vi "Main.vi"(11 "Module Admin":refnum<class "Delacor_lib_QMH_Module Admin.lvclass">) -> ()   [LabVIEW 2020, in "TCP_Server.lvlib"]
doc: "This template is based off of the Queued Message Handler design pattern and the Queued Message Handler project template that ships with LabVIEW.\n\nThe main difference is that the queue is private to this module and communication between modules is performed via Broadcast and Request events.\n\nRequest events are wrapped in public API methods and are handled in the Event Handling Loop (EHL) of this VI. Any module can register for Broadcast events sent by this module. The EHL generates messages based on user interface actions.\n\nThe Message Handling Loop (MHL) processes messages generated by the EHL, or by other messages. The messages are string values, so new messages can be added easily to the Message Cases case structure in the MHL. Each message cluster can also provide an optional value for Message Data, which is a variant that can be converted to whatever message-specific data is required.\n_____\nBased on DQMH Project Template 6.0.0.91."
uses:
  TCP_Server.lvlib
  <vilib>/Delacor/Delacor QMH/Libraries/Module Admin_class/Delacor_lib_QMH_Module Admin.lvclass
  Module Data--cluster.ctl
  <vilib>/Delacor/Delacor QMH/Libraries/Message Queue_class/Delacor_lib_QMH_Message Queue.lvclass/Delacor_lib_QMH_Message Queue.ctl
  Stop Argument--cluster.ctl
  <vilib>/Delacor/Delacor QMH/Libraries/Module Admin_class/Delacor_lib_QMH_Module Admin.lvclass/Delacor_lib_QMH_Module Admin.ctl
  <vilib>/Utility/miscctls.llb/LVPointTypeDef.ctl
  <vilib>/Delacor/Delacor QMH/Libraries/Message Queue_class/Delacor_lib_QMH_Enqueue Message (Single).vi
  <vilib>/Delacor/Delacor QMH/Libraries/Module Admin_class/Delacor_lib_QMH_Get External Launch.vi
  <vilib>/Utility/error.llb/Error Cluster From Error Code.vi
  <vilib>/ErrorRing/Error Ring.xnode
  <vilib>/Delacor/Delacor QMH/Libraries/Message Queue_class/Delacor_lib_QMH_Message Queue.lvclass
panel:
  out "concatenated string":string
  in  "Server":T1 {"Knob" scale=0.0..10.0; "Horizontal Fill Slide" scale=0.0..10.0}
  out "# of Connections":i32
  out "error out":errorcluster
  out "Status":string
  in  "Simulate MHL Error":bool
  in  "Simulate EHL Error":bool
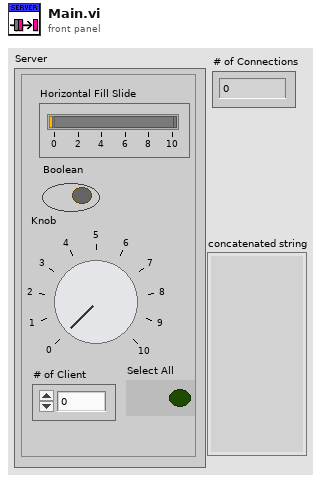
[diagram p1: front panel]
types:
  T1 = cluster{"Horizontal Fill Slide":dbl, "Knob":dbl, "Boolean":bool, "# of Client":i32, "Select All ":bool}
  T2 = typedef "TCP_Server.lvlib/Request Events--cluster.ctl" = cluster{"Stop Module":refnum<user-event>, "Show Panel":refnum<user-event>, "Hide Panel":refnum<user-event>, "Get Module Execution Status":refnum<user-event>, "Show Diagram":refnum<user-event>, "Wake Up HelperLoop":refnum<user-event>}
  T3 = typedef "TCP_Server.lvlib/Module Data--cluster.ctl" = cluster{"Status":string, "listener ID":refnum<k5>}
  T4 = enum32{"invalid lock state", "Not Locked", "Locked (No Password)", "Password-protected"}
  T5 = typedef "TCP_Server.lvlib/Stop Argument--cluster.ctl" = cluster{"Origin":string, "Exit via Stop Module Req?":bool, "Wait for Module to stop?":bool}
  T6 = typedef "LVPointTypeDef.ctl" = cluster{"Horizontal":i16, "Vertical":i16}
  T7 = enum32{"Invalid", "Standard", "Closed", "Hidden", "Minimized", "Maximized"}
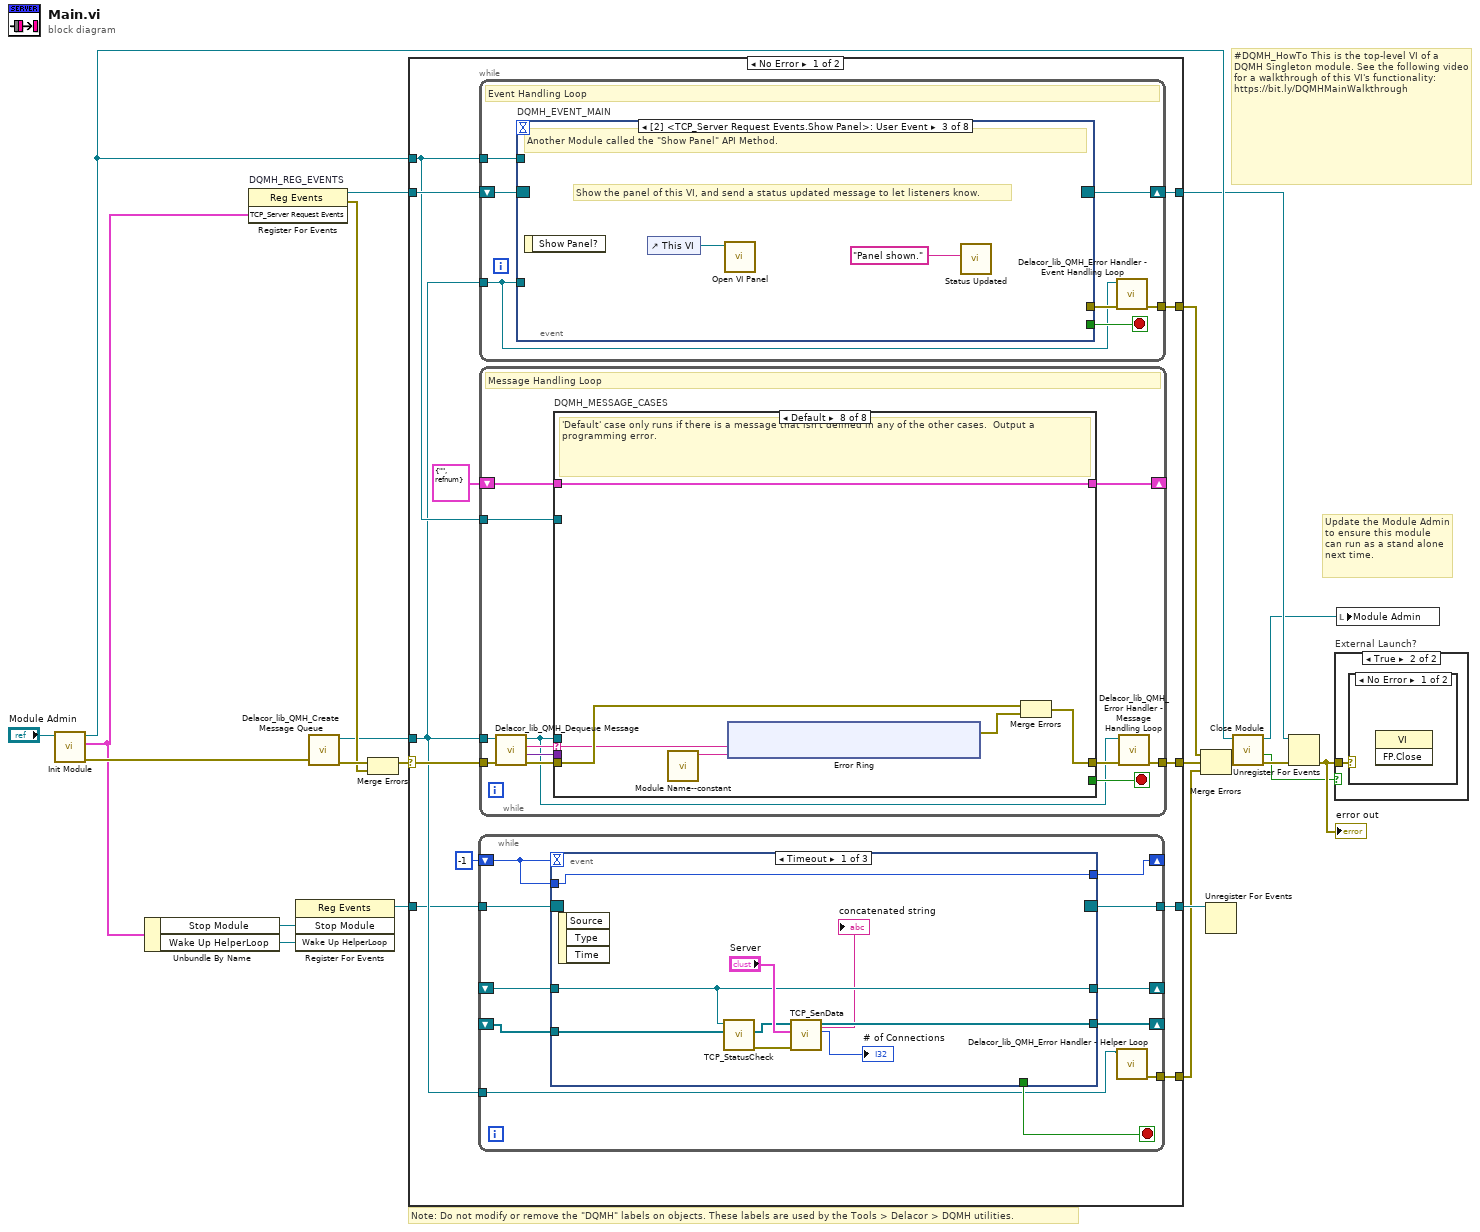
[diagram p0: block diagram]
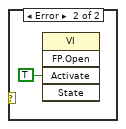
[diagram p3: hidden frame]
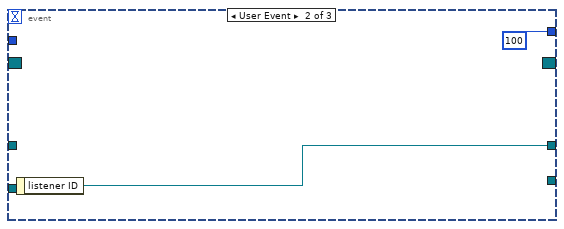
[diagram p4: hidden frame]
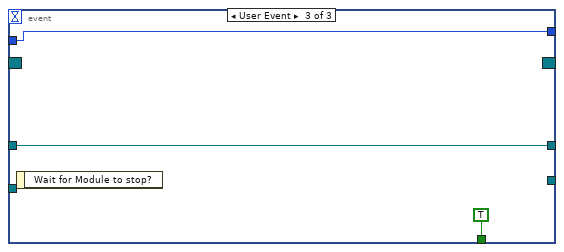
[diagram p5: hidden frame]
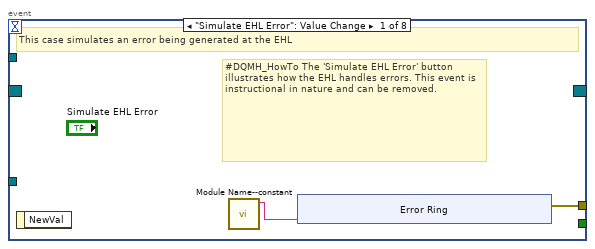
[diagram p6: hidden frame]
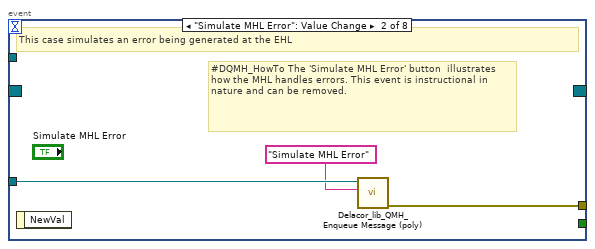
[diagram p7: hidden frame]
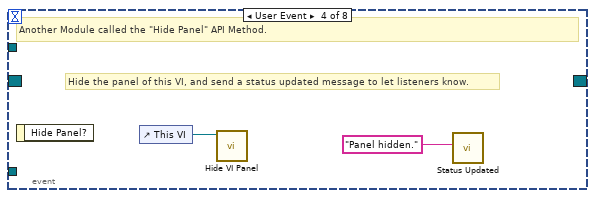
[diagram p8: hidden frame]
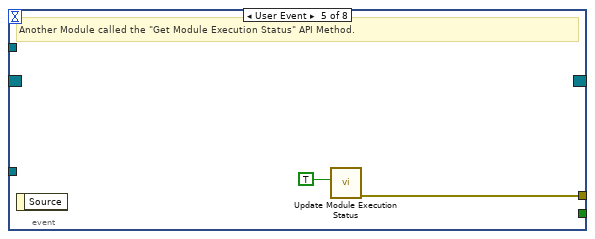
[diagram p9: hidden frame]
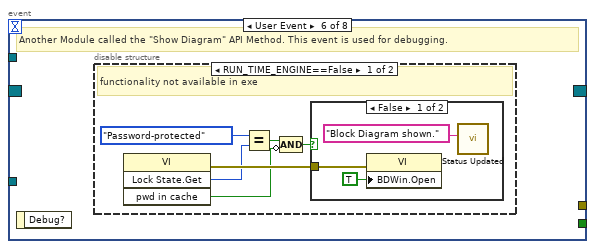
[diagram p10: hidden frame]
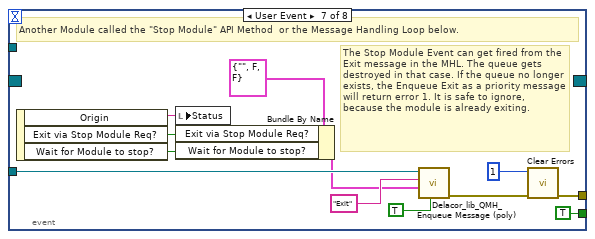
[diagram p13: hidden frame]
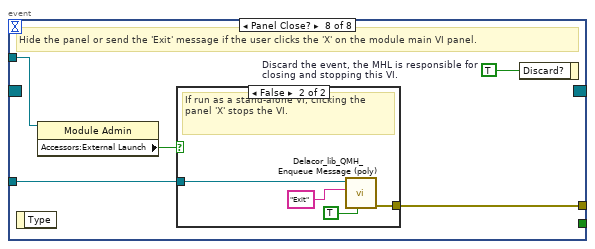
[diagram p14: hidden frame]
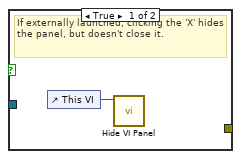
[diagram p15: hidden frame]
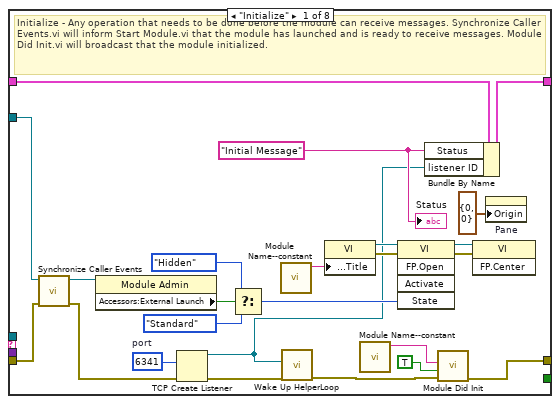
[diagram p16: hidden frame]
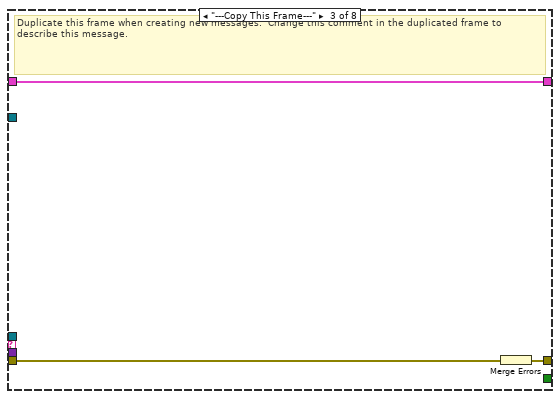
[diagram p18: hidden frame]
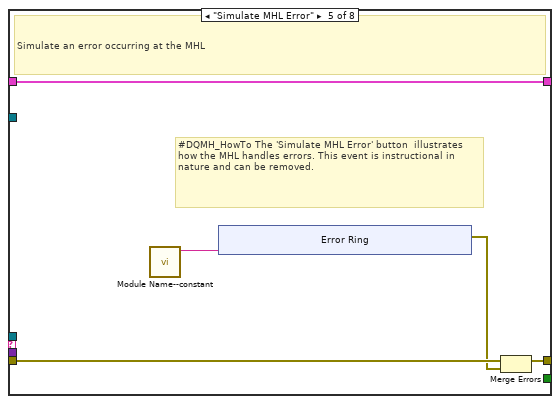
[diagram p20: hidden frame]
diagram:
  # "#DQMH_HowTo This is the top-level VI of a DQMH Singleton module. See the following video for a walkthrough of this VI's functionality: https://bit.ly/DQMHMainWalkthrough"
  # "Note: Do not modify or remove the \"DQMH\" labels on objects. These labels are used by the Tools > Delacor > DQMH utilities."
  # "Update the Module Admin to ensure this module can run as a stand alone next time."
  n1 = call "Init Module.vi"("Singleton Module Admin in"="Module Admin") -> ("error out"=w21:errorcluster, "TCP_Server Request Events"=w5:T2, "Singleton Module Admin out"=w13:refnum<class "Delacor_lib_QMH_Module Admin.lvclass">)  [unwired: 8 in]
  n2 = Unbundle By Name(w5) -> ("Stop Module"=w4:refnum<user-event>, "Wake Up HelperLoop"=w1:refnum<user-event>)
  n3 = register-events "DQMH_REG_EVENTS"(w5) -> (reference out=w11:refnum<event-registration>, error out=w14:errorcluster)  [unwired: 2 in]
  n4 = register-events(w4, w1) -> (reference out=w6:refnum<event-registration>)  [unwired: 2 in, 1 out]
  n5 = call <vilib>:"Delacor_lib_QMH_Create Message Queue.vi"("error in"=w21) -> ("error out"=w16:errorcluster, "Message Queue"=w10:refnum<class "Delacor_lib_QMH_Message Queue.lvclass">)  [unwired: 9 in]
  n6 = Merge Errors(w16, w14) -> (w15:errorcluster)
  n7 = case shown="No Error" w15 {
    selector: w15 -> [w32 w218]
    tunnel: [w34 w217] -> w22
    tunnel: [w31 w223] -> w12
    tunnel: w11 -> [w29 w223]
    tunnel: w10 -> [w27 w216]
    tunnel: [w33 _] -> w19
    tunnel: w13 -> [w28 w219]
    tunnel: w6 -> [w26 _]
    tunnel: [w24 _] -> w3
    tunnel: [w23 _] -> w2
    frame No Error {
      n8 = while {
        tunnel: w27 -> [w40]
        tunnel: w26 -> [w45]
        shift-right: [w43] -> _
        shift-left: -1 -> [w44]
        tunnel: [w42] -> w24
        tunnel: [w39] -> w23
        shift-right: [w38] -> _
        shift-left: _ -> [w37]
        shift-right: [w36] -> _
        shift-left: _ -> [w35]
        stop <- w41 stop-if-true
        n9 = event shown="[0] Timeout" {
          selector: w45 -> [_ _ _]
          dyn-events: [_ _ _] -> w42
          timeout: w44 -> [_ _ _]
          tunnel: w44 -> [w54 _ w57]
          tunnel: [w54 100 w57] -> w43
          tunnel: [_ _ TRUE] -> w41
          tunnel: [w47 w55 w58] -> w38
          tunnel: w37 -> [w47 _ w58]
          tunnel: [w52 _ _] -> w36
          tunnel: w35 -> [w48 _ _]
          event Timeout {
            n10 = event-data() -> ()  [unwired: 1 in, 3 out]
            n11 = call "TCP_StatusCheck.vi"("Clients"=w48, "listener ID in"=w47) -> ("no error"=w53:errorcluster, "Clients"=w49:refnum<k5>[])  [unwired: 7 in, 1 out]
            n12 = call "TCP_SenData.vi"("error in"=w53, "Server"="Server", "Clients"=w49) -> ("# of Connections"=→"# of Connections":i32, "Clients"=w52:refnum<k5>[], "concatenated string"=→"concatenated string":string)  [unwired: 4 in, 2 out]
          }
          event User Event {
            n13 = event-data() -> ("listener ID"=w55:refnum<k5>)  [unwired: 1 in]
          }
          event User Event {
            n14 = event-data() -> ()  [unwired: 1 in, 1 out]
          }
        }
        n15 = call-dynamic "Delacor_lib_QMH_Error Handler - Helper Loop.vi"("Message Queue in"=w40) -> ("dup error in"=w39:errorcluster)  [unwired: 9 in, 1 out]
      }
      n16 = while {
        tunnel: w27 -> [w60]
        shift-right: [w63] -> w31
        shift-left: w29 -> [w64]
        tunnel: [w65] -> w33
        tunnel: w28 -> [w61]
        stop <- w62 stop-if-true
        # "Event Handling Loop"
        n17 = event "DQMH_EVENT_MAIN" shown="[2] <TCP_Server Request Events.Show Panel>: User Event" {
          selector: w64 -> [_ _ _ _ _ _ _ _]
          dyn-events: [_ _ _ _ _ _ _ _] -> w63
          timeout: _ -> [_ _ _ _ _ _ _ _]
          tunnel: [_ _ _ _ _ _ TRUE ("Discard?") _] -> w62
          tunnel: w60 -> [_ w77 _ _ _ _ w101 w108]
          tunnel: [w68 w78 _ _ w84 _ w104 w110] -> w66
          tunnel: w61 -> [_ _ _ _ _ _ _ w107]
          event "Simulate EHL Error": Value Change {
            # "#DQMH_HowTo The 'Simulate EHL Error' button  illustrates how the EHL handles errors. This event is instructional in nature and can be removed."
            # "This case simulates an error being generated at the EHL"
            n18 = event-data() -> ()  [unwired: 1 in, 1 out]
            n19 = call "Module Name--constant.vi"() -> ("Module Name"=w67:string)  [unwired: 11 in]
            n20 = xnode "Error Ring"("parameter 0"=w67) -> ("error out"=w68:errorcluster)
          }
          event "Simulate MHL Error": Value Change {
            # "#DQMH_HowTo The 'Simulate MHL Error' button  illustrates how the MHL handles errors. This event is instructional in nature and can be removed."
            # "This case simulates an error being generated at the EHL"
            n21 = event-data() -> ()  [unwired: 1 in, 1 out]
            n22 = call-poly <vilib>:"Delacor_lib_QMH_Enqueue Message (poly).vi"("Message"="Simulate MHL Error", "Message Queue in"=w77) -> ("error out"=w78:errorcluster)  [unwired: 8 in, 1 out]
          }
          event User Event {
            # "Show the panel of this VI, and send a status updated message to let listeners know."
            # "Another Module called the \"Show Panel\" API Method."
            n23 = event-data() -> ()  [unwired: 1 in, 1 out]
            n24 = control-ref of="This VI"() -> (w80:refnum<vi>)
            n25 = call "Open VI Panel.vi"("VI"=w80) -> ()  [unwired: 10 in, 1 out]
            n26 = call "Status Updated.vi"("Status"="Panel shown." ("format string")) -> ()  [unwired: 10 in, 1 out]
          }
          event User Event {
            # "Hide the panel of this VI, and send a status updated message to let listeners know."
            # "Another Module called the \"Hide Panel\" API Method."
            n27 = event-data() -> ()  [unwired: 1 in, 1 out]
            n28 = control-ref of="This VI"() -> (w82:refnum<vi>)
            n29 = call "Hide VI Panel.vi"("VI"=w82) -> ()  [unwired: 10 in, 1 out]
            n30 = call "Status Updated.vi"("Status"="Panel hidden." ("format string")) -> ()  [unwired: 10 in, 1 out]
          }
          event User Event {
            # "Another Module called the \"Get Module Execution Status\" API Method."
            n31 = event-data() -> ()  [unwired: 1 in, 1 out]
            n32 = call "Update Module Execution Status.vi"("Running?"=TRUE) -> ("error out"=w84:errorcluster)  [unwired: 10 in]
          }
          event User Event {
            # "Another Module called the \"Show Diagram\" API Method. This event is used for debugging."
            n33 = event-data() -> ()  [unwired: 1 in, 1 out]
            n34 = disable-structure shown="RUN_TIME_ENGINE==False" {
              frame condition #0 (active) {
                # "functionality not available in exe"
                n35 = invoke class="VI" method="Lock State.Get"() -> (error out=w90:errorcluster, "Get Lock State"=w89:T4, "pwd in cache"=w86:bool)  [unwired: 4 in, 1 out]
                n36 = Equal?(x=T4."Password-protected", y=w89) -> (x = y?=w87:bool)
                n37 = Compound Arithmetic op=AND(w87, invert w86) -> (w85:bool)
                n38 = case shown="False" w85 {
                  tunnel: w90 -> [w93 _]
                  frame False {
                    n39 = property class="VI"(error in=w93, "BDWin.Open"=TRUE ("Block Diagram Window:Open")) -> ()  [unwired: 1 in, 2 out]
                    n40 = call "Status Updated.vi"("Status"="Block Diagram shown." ("format string")) -> ()  [unwired: 10 in, 1 out]
                  }
                  frame True {
                    # "Password-protected VI, and the password is not in the cache. Do not show the diagram."
                  }
                }
              }
              frame condition #1 {
              }
            }
          }
          event User Event {
            # "The Stop Module Event can get fired from the Exit message in the MHL. The queue gets destroyed in that case. If the queue no longer exists, the Enqueue Exit as a priority message will return error 1. It is safe to ignore, because the module is already exiting."
            # "Another Module called the \"Stop Module\" API Method  or the Message Handling Loop below."
            n41 = event-data() -> ("Origin"=w100:string, "Exit via Stop Module Req?"=w96:bool, "Wait for Module to stop?"=w95:bool)  [unwired: 1 in]
            n42 = local write "Status"(w100) -> ()
            n43 = Bundle By Name(cluster=T5 {"Origin"="", "Exit via Stop Module Req?"=FALSE, "Wait for Module to stop?"=FALSE} ("Stop Argument"), "Exit via Stop Module Req?"=w96, "Wait for Module to stop?"=w95) -> (w94:T5)
            n44 = call-poly <vilib>:"Delacor_lib_QMH_Enqueue Message (poly).vi"("Priority Message? (F)"=TRUE, "Message Data"=w94, "Message"="Exit", "Message Queue in"=w101) -> ("error out"=w105:errorcluster)  [unwired: 6 in, 1 out]
            n45 = call <vilib>:"Clear Errors.vi"("error in (no error)"=w105, "specific error code to clear (0: all)"=1) -> ("error out"=w104:errorcluster)  [unwired: 4 in, 1 out]
          }
          event Panel Close? {
            w109 = TRUE  # Discard the event, the MHL is responsible for closing and stopping this VI.
            # "Hide the panel or send the 'Exit' message if the user clicks the 'X' on the module main VI panel."
            n46 = event-data() -> ()  [unwired: 1 in, 1 out]
            n47 = property class="Module Admin"(reference=w107) -> ("Accessors:External Launch"=w106:bool)  [unwired: 1 in, 2 out]
            n48 = case shown="False" w106 {
              tunnel: w108 -> [_ w114]
              tunnel: [_ w115] -> w110
              frame True {
                # "If externally launched, clicking the 'X' hides the panel, but doesn't close it."
                n49 = control-ref of="This VI"() -> (w111:refnum<vi>)
                n50 = call "Hide VI Panel.vi"("VI"=w111) -> ()  [unwired: 10 in, 1 out]
              }
              frame False {
                # "If run as a stand-alone VI, clicking the panel 'X' stops the VI."
                n51 = call-poly <vilib>:"Delacor_lib_QMH_Enqueue Message (poly).vi"("Priority Message? (F)"=TRUE, "Message"="Exit", "Message Queue in"=w114) -> ("error out"=w115:errorcluster)  [unwired: 7 in, 1 out]
              }
            }
            n52 = event-data("Discard?"=w109) -> ()  [unwired: 1 in, 1 out]
          }
        }
        n53 = call-dynamic "Delacor_lib_QMH_Error Handler - Event Handling Loop.vi"("error in"=w66, "Message Queue in"=w60) -> ("dup error in"=w65:errorcluster)  [unwired: 8 in, 1 out]
      }
      n54 = while {
        tunnel: w27 -> [w118]
        shift-right: [w122] -> _
        shift-left: T3 {"Status"="", "listener ID"=refnum} ("Data Cluster") -> [w123]
        tunnel: w32 -> [w126]
        tunnel: [w124] -> w34
        tunnel: w28 -> [w116]
        stop <- w121 stop-if-true
        # "Message Handling Loop"
        n55 = call-dynamic "Delacor_lib_QMH_Dequeue Message.vi"("error in"=w126, "Message Queue in"=w118) -> ("error out"=w125:errorcluster, "Message Data"=w119:variant, "Message"=w120:string, "Message Queue out"=w117:refnum<class "Delacor_lib_QMH_Message Queue.lvclass">)  [unwired: 6 in]
        n56 = case "DQMH_MESSAGE_CASES" shown="Default" w120 {
          selector: w120 -> [_ _ _ _ _ _ _ w203]
          tunnel: w117 -> [_ _ _ _ _ w173 w195 _]
          tunnel: w125 -> [w149 w153 w156 w158 w163 w180 w201 w205]
          tunnel: [w148 w153 w155 w158 w162 w176 w198 w206] -> w127
          tunnel: w123 -> [w139 w152 w154 w157 w160 w175 w194 w204]
          tunnel: [w138 w152 w154 w157 w160 w175 w194 w204] -> w122
          tunnel: [_ _ _ _ _ _ w193 _] -> w121
          tunnel: w119 -> [_ _ _ _ _ w174 w192 _]
          tunnel: w116 -> [w140 _ _ _ _ w172 w187 _]
          frame "Initialize" {
            w131 = u16 6341  # port
            w134 = "Initial Message" ("Initial Message")
            # "Initialize - Any operation that needs to be done before the module can receive messages. Synchronize Caller Events.vi will inform Start Module.vi that the module has launched and is ready to receive messages. Module Did Init.vi will broadcast that the module initialized."
            n57 = call "Synchronize Caller Events.vi"("error in (no error)"=w149, "Singleton Module Admin in"=w140) -> ("error out"=w132:errorcluster, "Singleton Module Admin out"=w135:refnum<class "Delacor_lib_QMH_Module Admin.lvclass">)  [unwired: 8 in]
            n58 = property class="Module Admin"(reference=w135) -> ("Accessors:External Launch"=w144:bool)  [unwired: 1 in, 2 out]
            n59 = TCP Create Listener(8:w132, 10:w131) -> (0:w130:errorcluster, 3:w128:refnum<k5>)  [unwired: 1 in, 3 out]
            n60 = Select(t=T7."Hidden" ("State"), s=w144, f=T7."Standard" ("State")) -> (s? t:f=w141:T7)
            n61 = call "Module Name--constant.vi"() -> ("Module Name"=w147:string)  [unwired: 11 in]
            n62 = call "Wake Up HelperLoop.vi"("error in"=w130, "listener ID"=w128) -> ("error out"=w129:errorcluster)  [unwired: 9 in]
            n63 = property class="VI"("Front Panel.Title"=w147) -> (reference out=w146:refnum<vi>, error out=w151:errorcluster)  [unwired: 2 in]
            n64 = call "Module Name--constant.vi"() -> ("Module Name"=w136:string)  [unwired: 11 in]
            n65 = invoke class="VI" method="FP.Open"(reference=w146, error in=w151, "State"=w141) -> (reference out=w145:refnum<vi>, error out=w150:errorcluster)  [unwired: 2 in, 3 out]
            n66 = Bundle By Name(cluster=w139, "Status"=w134, "listener ID"=w128) -> (w138:T3)
            n67 = call "Module Did Init.vi"("error in (no error)"=w129, "Initialized?"=TRUE, "Origin"=w136) -> ("error out"=w148:errorcluster)  [unwired: 8 in]
            n68 = invoke class="VI" method="FP.Center"(reference=w145, error in=w150) -> ()  [unwired: 1 in, 3 out]
            n69 = property on="Pane" class="Pane"("Origin"=T6 {"Horizontal"=0, "Vertical"=0}) -> ()  [unwired: 2 in, 2 out]
            "Status" <- w134
          }
          frame "---Module Specific---" {
            # "Separator -- The following cases handle messages specific to this Module."
          }
          frame "---Copy This Frame---" {
            # "Duplicate this frame when creating new messages.  Change this comment in the duplicated frame to describe this message."
            n70 = Merge Errors(w156) -> (w155:errorcluster)
          }
          frame "---Exit and Error Handling---" {
            # "Separator - The following cases handle errors and exit messages."
          }
          frame "Simulate MHL Error" {
            # "#DQMH_HowTo The 'Simulate MHL Error' button  illustrates how the MHL handles errors. This event is instructional in nature and can be removed."
            # "Simulate an error occurring at the MHL"
            n71 = call "Module Name--constant.vi"() -> ("Module Name"=w159:string)  [unwired: 11 in]
            n72 = xnode "Error Ring"("parameter 0"=w159) -> ("error out"=w161:errorcluster)
            n73 = Merge Errors(w163, w161) -> (w162:errorcluster)
          }
          frame "Error" {
            # "#CodeRecommended - If you ever change the name of this \"Error\" message, you'll need to update the name in the Check Loop Error.vi as well."
            # "#CodeRecommended - If the module is running in standalone mode (External Launch = FALSE), this code will pop up an error dialog and call the 'Exit' message if an error occurs. Add more fine-grained error handling here."
            # "Error - Check the error message data and respond accordingly. This message is sent by the \"Error Handler\" VIs at the end of each loop in this application."
            n74 = property class="Module Admin"(reference=w172) -> ("Accessors:External Launch"=w171:bool)  [unwired: 1 in, 2 out]
            n75 = Variant To Data(error in=w180, type=errorcluster {"status"=FALSE, "code"=0, "source"=""} ("error constant"), Variant=w174) -> (data=w181:errorcluster, error out=w178:errorcluster)
            n76 = call "Error Reported.vi"("Error"=w181) -> ()  [unwired: 10 in, 1 out]
            n77 = case shown="False" w171 {
              tunnel: [w186 _] -> w177
              tunnel: w173 -> [w184 _]
              tunnel: w181 -> [w185 _]
              frame False {
                # "If the module is running standalone, then pop up an error dialog and call the \"Exit\" message."
                n78 = call <vilib>:"Simple Error Handler.vi"("error in (no error)"=w185) -> ()  [unwired: 4 in, 5 out]
                n79 = call-poly <vilib>:"Delacor_lib_QMH_Enqueue Message (poly).vi"("Priority Message? (F)"=TRUE, "Message"="Exit", "Message Queue in"=w184) -> ("error out"=w186:errorcluster)  [unwired: 7 in, 1 out]
              }
              frame True {
                # "If the module was launched externally, calling the Error Reported broadcast VI is the only action performed by the \"Error\" message. The module's caller can then process the error appropriately."
              }
            }
            n80 = Merge Errors(w178, w177) -> (w176:errorcluster)
            n81 = local write "error out"(w176) -> ()
          }
          frame "Exit" {
            w191 = 91  # 91: not all Exit messages will have an argument
            w193 = TRUE  # Stop the VI
            # "Release the message queue reference"
            # "#CodeNeeded - Add any required cleanup code here"
            # "Exit - Exit the application."
            n82 = Variant To Data(error in=w201, type=T5 {"Origin"="", "Exit via Stop Module Req?"=FALSE, "Wait for Module to stop?"=FALSE} ("Stop Argument"), Variant=w192) -> (data=w189:T5, error out=w197:errorcluster)
            n83 = call <vilib>:"Clear Errors.vi"("error in (no error)"=w197, "specific error code to clear (0: all)"=w191) -> ("error out"=w200:errorcluster)  [unwired: 4 in, 1 out]
            n84 = control-ref of="This VI"() -> (w188:refnum<vi>)
            n85 = call-dynamic "Delacor_lib_QMH_Release Message Queue.vi"("error in"=w200, "Message Queue"=w195) -> ("error out"=w199:errorcluster)  [unwired: 9 in]
            n86 = call "Handle Exit.vi"("Stop Argument"=w189, "Admin in"=w187, "VI reference"=w188) -> ("error out"=w196:errorcluster)  [unwired: 7 in, 1 out]
            n87 = Merge Errors(w199, w196) -> (w198:errorcluster)
          }
          frame Default {
            # "'Default' case only runs if there is a message that isn't defined in any of the other cases.  Output a programming error."
            n88 = call "Module Name--constant.vi"() -> ("Module Name"=w202:string)  [unwired: 11 in]
            n89 = xnode "Error Ring"("parameter 0"=w203, "parameter 1"=w202) -> ("error out"=w207:errorcluster)
            n90 = Merge Errors(w205, w207) -> (w206:errorcluster)
          }
        }
        n91 = call-dynamic "Delacor_lib_QMH_Error Handler - Message Handling Loop.vi"("error in"=w127, "Message Queue in"=w117) -> ("dup error in"=w124:errorcluster)  [unwired: 8 in, 1 out]
      }
    }
    frame Error {
      # "Synchronize Caller Events.vi will inform Start Module.vi that the module has launched and will let the code calling Start Module.vi register for broadcasts and would permit the caller receive the broadcast that an error occurred at launch time."
      n92 = call-dynamic "Delacor_lib_QMH_Release Message Queue.vi"("error in"=w218, "Message Queue"=w216) -> ("error out"=w217:errorcluster)  [unwired: 9 in]
      n93 = call "Synchronize Caller Events.vi"("Singleton Module Admin in"=w219) -> ("error out"=w224:errorcluster)  [unwired: 9 in, 1 out]
      n94 = call "Module Name--constant.vi"() -> ("Module Name"=w222:string)  [unwired: 11 in]
      n95 = Format Into String(format string="An error occurred during initialization. %s is no longer running.", w222) -> (resulting string=w220:string)  [unwired: 2 in, 1 out]
      n96 = Merge Errors(w217, w224) -> (w225:errorcluster)
      n97 = call "Error Reported.vi"("Additional Information"=w220, "Error"=w225) -> ()  [unwired: 9 in, 1 out]
    }
  }
  n98 = Merge Errors(w19, w22, w2) -> (w18:errorcluster)
  n99 = Unregister For Events(event registration refnum=w3) -> ()  [unwired: 1 in, 1 out]
  n100 = call "Close Module.vi"("error in (no error)"=w18, "Module Admin in"=w13) -> ("error out"=w20:errorcluster, "External Launch"=w7:bool, "Module Admin out"=w8:refnum<class "Delacor_lib_QMH_Module Admin.lvclass">)  [unwired: 7 in]
  n101 = Unregister For Events(event registration refnum=w12, error in=w20) -> (error out=w17:errorcluster)
  "error out" <- w17
  n102 = case "External Launch?" shown="True" w7 {
    tunnel: w17 -> [_ w226]
    frame False {
    }
    frame True {
      n103 = case shown="No Error" w226 {
        frame No Error {
          n104 = invoke class="VI" method="FP.Close"() -> ()  [unwired: 3 in, 3 out]
        }
        frame Error {
          n105 = invoke class="VI" method="FP.Open"("Activate"=TRUE ("Activate?")) -> ()  [unwired: 4 in, 5 out]
        }
      }
    }
  }
  n106 = local write "Module Admin"(w8) -> ()
